vi "createNetCostMatrix.vi"(8 "error in (no error)":errorcluster, 10 "Edges":T1(array[cluster]), 11 "Number of Nodes":i32) -> (0 "error out":errorcluster, 3 "netCostMatrix":dbl[][](array[numeric]))   [LabVIEW 2009]
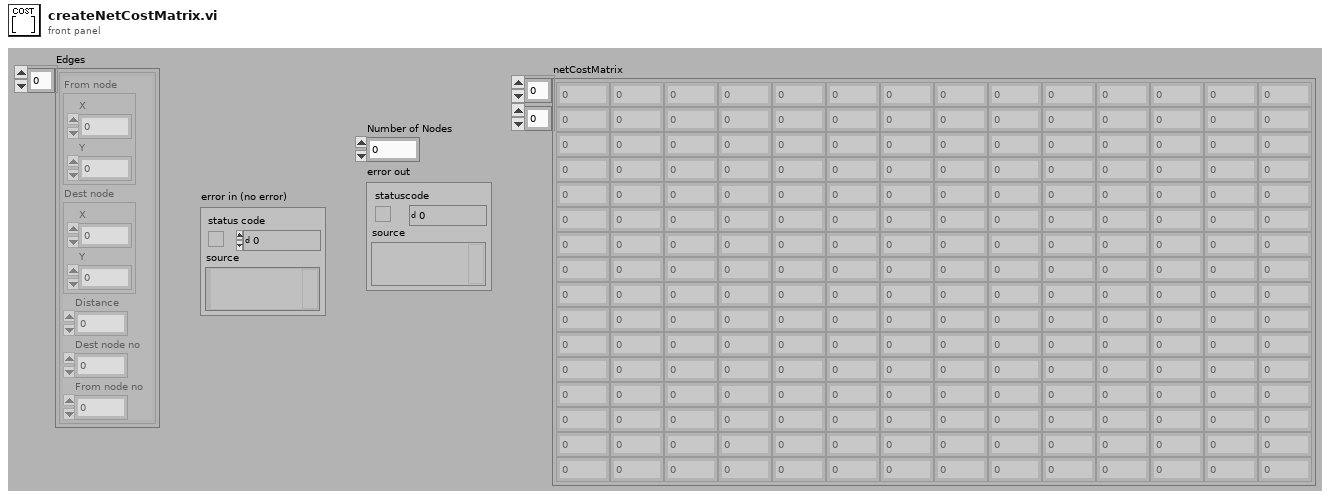
[diagram p1: front panel]
types:
  T1 = cluster{"From node":cluster{"X":dbl, "Y":dbl}, "Dest node":cluster{"X":dbl, "Y":dbl}, "Distance":dbl, "Dest node no":i32, "From node no":i32}[]
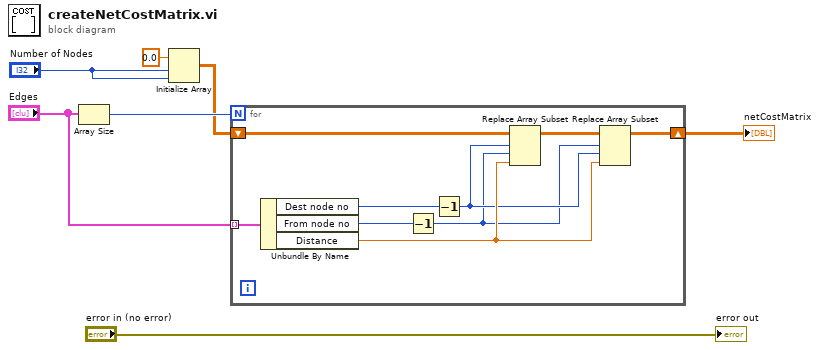
[diagram p0: block diagram]
diagram:
  n1 = Array Size(array="Edges") -> (size(s)=w6:i32)
  n2 = Initialize Array(0.0 ("element"), "Number of Nodes", "Number of Nodes") -> (w4:dbl[][])
  n3 = for {
    N: w6 -> [_]
    tunnel: "Edges" -> [w16] mode=indexing
    shift-right: [w12] -> w3
    shift-left: w4 -> [w15]
    n4 = Unbundle By Name(w16) -> ("Dest node no"=w10:i32, "From node no"=w8:i32, "Distance"=w13:dbl)
    n5 = Decrement(x=w8) -> (x-1=w9:i32)
    n6 = Decrement(x=w10) -> (x-1=w11:i32)
    n7 = Replace Array Subset(array=w15, new element=w13, index (row)=w11, index (col)=w9) -> (w14:dbl[][])
    n8 = Replace Array Subset(array=w14, new element=w13, index (row)=w9, index (col)=w11) -> (w12:dbl[][])
  }
  "netCostMatrix" <- w3
  "error out" <- "error in (no error)"
